vi "Init.vi"(8 "error in (no error)":errorcluster, 9 "Simulated/real":bool, 10 "cameras quantity":u8, 11 "Channel Manager in":refnum<class "Channel Manager.lvclass">) -> (0 "error out":errorcluster, 3 "Channel Manager out":refnum<class "Channel Manager.lvclass">)   [LabVIEW 2018, in "Channel Manager.lvclass"]
uses:
  Channel Manager.lvclass
  Channel/Channel.lvclass
  Channel Manager.lvclass/Channel Manager.ctl
panel:
  in  "Channel.lvclass":refnum<class "Channel.lvclass">
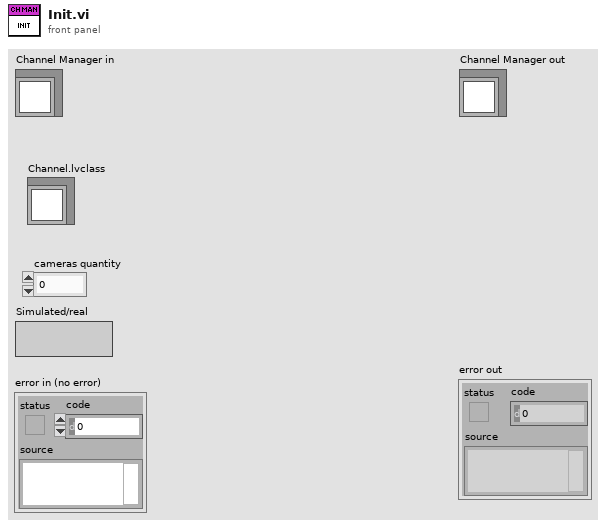
[diagram p1: front panel]
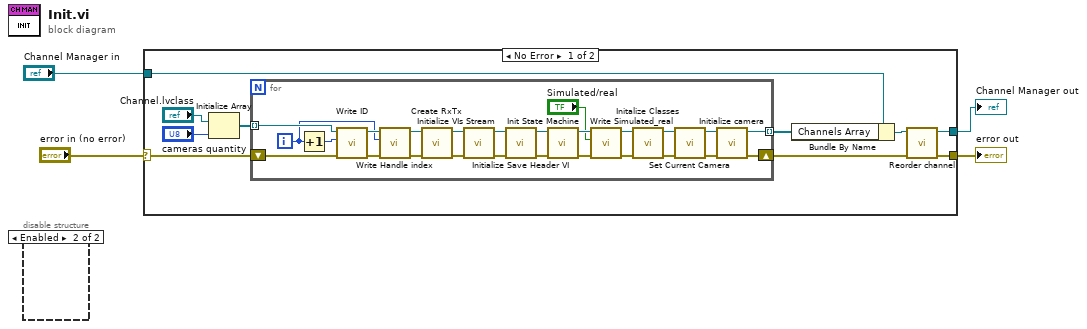
[diagram p0: block diagram]
diagram:
  n1 = disable-structure shown="Enabled" {
    frame Disabled {
    }
    frame Enabled {
    }
  }
  n2 = case shown="No Error" "error in (no error)" {
    selector: "error in (no error)" -> [w14 w41]
    tunnel: [w8 w41] -> w3
    tunnel: [w9 w40] -> w1
    tunnel: "Channel Manager in" -> [w12 w40]
    frame No Error {
      n3 = Initialize Array("Channel.lvclass", "cameras quantity") -> (w7:refnum<class "Channel.lvclass">[])
      n4 = for {
        tunnel: w7 -> [w37] mode=indexing
        tunnel: [w27] -> w6 mode=indexing
        shift-right: [w28] -> w5
        shift-left: w14 -> [w36]
        i -> [w19]
        n5 = Increment(x=w19) -> (x+1=w35:i32)
        n6 = call "Write ID.vi"("error in (no error)"=w36, "ID"=w35, "Channel in"=w37) -> ("error out"=w24:errorcluster, "Channel out"=w25:refnum<class "Channel.lvclass">)  [unwired: 7 in]
        n7 = call "Write Handle index.vi"("error in (no error)"=w24, "Handle index"=w19, "Channel in"=w25) -> ("error out"=w23:errorcluster, "Channel out"=w22:refnum<class "Channel.lvclass">)  [unwired: 7 in]
        n8 = call "Create RxTx.vi"("error in (no error)"=w23, "Channel in"=w22) -> ("error out"=w38:errorcluster, "Channel out"=w39:refnum<class "Channel.lvclass">)  [unwired: 8 in]
        n9 = call "Initialize VIs Stream.vi"("error in (no error)"=w38, "Channel in"=w39) -> ("error out"=w15:errorcluster, "Channel out"=w18:refnum<class "Channel.lvclass">)  [unwired: 8 in]
        n10 = call "Initialize Save Header VI.vi"("error in (no error)"=w15, "Channel in"=w18) -> ("error out"=w16:errorcluster, "Channel out"=w17:refnum<class "Channel.lvclass">)  [unwired: 8 in]
        n11 = call "Init State Machine.vi"("error in (no error)"=w16, "Channel in"=w17) -> ("error out"=w29:errorcluster, "Channel out"=w30:refnum<class "Channel.lvclass">)  [unwired: 8 in]
        n12 = call "Write Simulated_real.vi"("error in (no error)"=w29, "Simulated/real"="Simulated/real", "Channel in"=w30) -> ("error out"=w20:errorcluster, "Channel out"=w21:refnum<class "Channel.lvclass">)  [unwired: 7 in]
        n13 = call "Initalize Classes.vi"("error in (no error)"=w20, "Channel in"=w21) -> ("error out"=w32:errorcluster, "Channel out"=w31:refnum<class "Channel.lvclass">)  [unwired: 8 in]
        n14 = call "Set Current Camera.vi"("error in (no error)"=w32, "Channel in"=w31) -> ("error out"=w34:errorcluster, "Channel out"=w33:refnum<class "Channel.lvclass">)  [unwired: 8 in]
        n15 = call "Initialize camera.vi"("error in (no error)"=w34, "Channel in"=w33) -> ("error out"=w28:errorcluster, "Channel out"=w27:refnum<class "Channel.lvclass">)  [unwired: 8 in]
      }
      n16 = Bundle By Name(cluster=w12, "Channels Array"=w6) -> (w10:refnum<class "Channel Manager.lvclass">)
      n17 = call "Reorder channel.vi"("error in (no error)"=w5, "Channel Manager in"=w10) -> ("error out"=w8:errorcluster, "Channel Manager out"=w9:refnum<class "Channel Manager.lvclass">)  [unwired: 8 in]
    }
    frame Error {
    }
  }
  "error out" <- w3
  "Channel Manager out" <- w1
